vi "graph_temp.vi"(9 "Termistor":dbl format="%#.2g", 10 "Array":cluster{"Time":timestamp, "Data":dbl}[](array[cluster])) -> (2 "XY Graph":cluster{"Time":timestamp, "Data":dbl}[](graph))   [LabVIEW 2010]
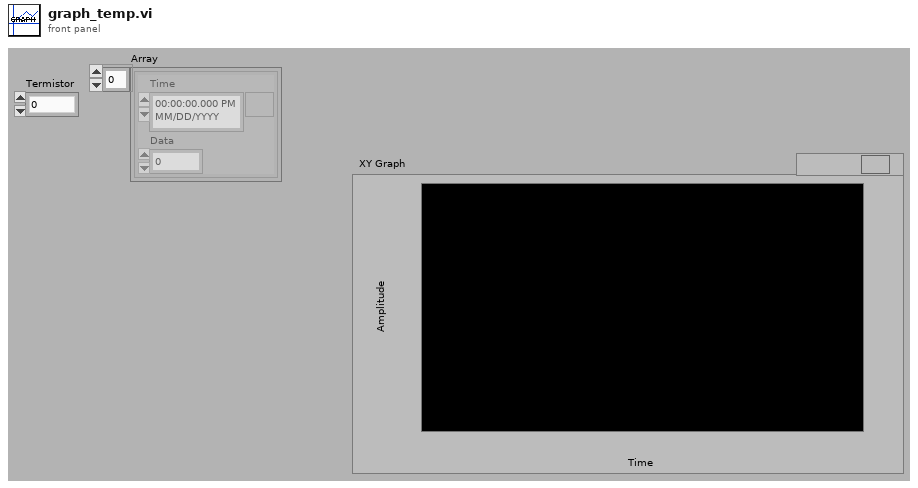
[diagram p1: front panel]
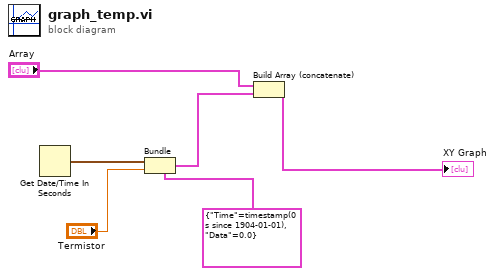
[diagram p0: block diagram]
diagram:
  n1 = Get Date/Time In Seconds() -> (seconds since 1Jan1904=w4:timestamp)
  n2 = Bundle(cluster=cluster{"Time":timestamp, "Data":dbl} {"Time"=timestamp(0 s since 1904-01-01), "Data"=0.0}, "Time"=w4, "Data"="Termistor") -> (w5:cluster{"Time":timestamp, "Data":dbl})
  n3 = Build Array (concatenate)("Array", w5) -> (→"XY Graph":cluster{"Time":timestamp, "Data":dbl}[])
